vi "RW_Module.vi"(7 "N_modules":i32, 8 "error in":errorcluster, 9 "RD_WR param":T1, 10 "Data Reference":T2, 11 "Status Reference":T3) -> (0 "error out":errorcluster, 1 "stopped":bool)   [LabVIEW 2019, in "MB_TCP1.lvlib"]
uses:
  MB_TCP1.lvlib
  ICPCON Status/Ctl/ICPCON Status.ctl
  ICPCON Registers/Ctl/ICPCON Data.ctl
  ICPCON Param/ICPCON Param.ctl
  MB_TCP_NS300.vi
  MB_TCP_7016i.vi
  MB_TCP_7051.vi
  MB_TCP_7024i.vi
  MB_TCP_7018o.vi
  MB_TCP_7018.vi
  MB_TCP_7018i.vi
  MB_TCP_7017.vi
  MB_TCP_ZERO.vi
  ICPCON Status/ICPCON Status.lvlib
  ICPCON Registers/ICPCON Registers.lvlib
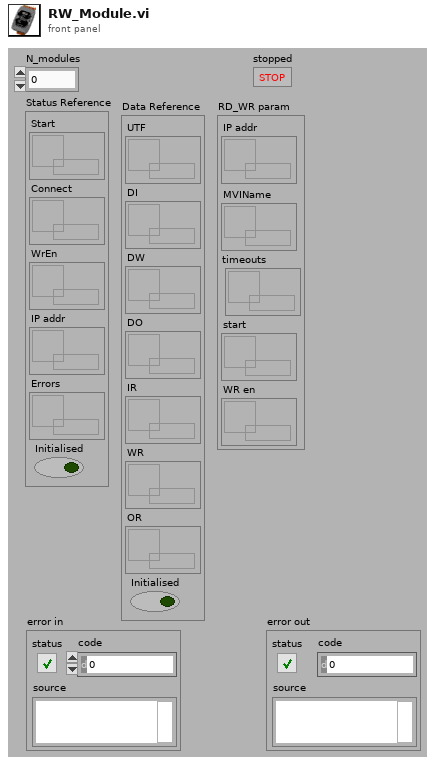
[diagram p1: front panel]
types:
  T1 = typedef "ICPCON Param.ctl" = cluster{"IP addr":refnum<data-value>, "MVIName":refnum<data-value>, "timeouts":refnum<data-value>, "start":refnum<data-value>, "WR en":refnum<data-value>}
  T2 = typedef "ICPCON Registers.lvlib/ICPCON Data.ctl" = cluster{"UTF":refnum<data-value>, "DI":refnum<data-value>, "DW":refnum<data-value>, "DO":refnum<data-value>, "IR":refnum<data-value>, "WR":refnum<data-value>, "OR":refnum<data-value>, "Initialised":bool}
  T3 = typedef "ICPCON Status.lvlib/ICPCON Status.ctl" = cluster{"Start":refnum<data-value>, "Connect":refnum<data-value>, "WrEn":refnum<data-value>, "IP addr":refnum<data-value>, "Errors":refnum<data-value>, "Initialised":bool}
  T4 = enum16{"initialize", "call modules", "work", "stop modules", "standby"}
  T5 = enum32{"Bad", "Idle", "Run top level", "Running"}
  T6 = cluster{"Remote IP Address":string, "Remote Port":u16}[]
  T7 = cluster{"conn_timeout":i32, "reconn_timeout":i32, "N attempt max":i32, "t_reset_TTL":i32, "write_timeout":i32, "read_timeout":i32, "period":i32}[]
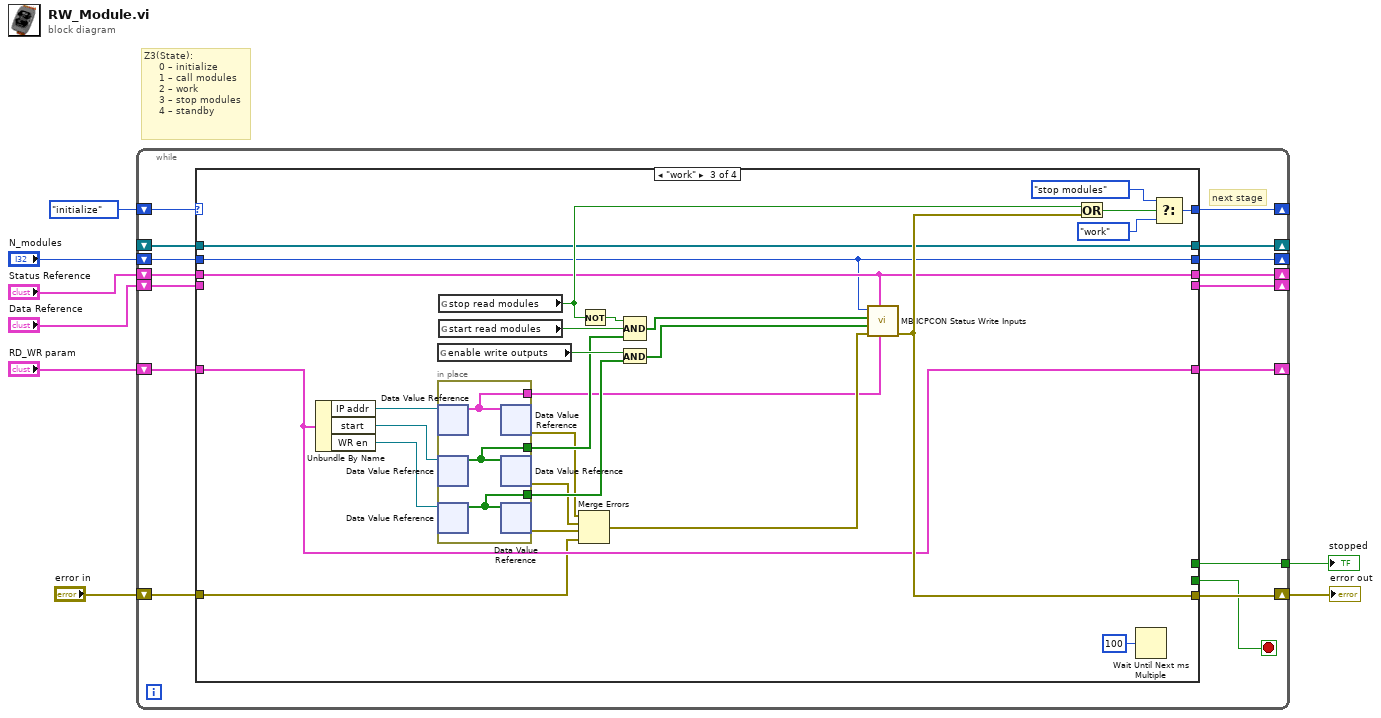
[diagram p0: block diagram]
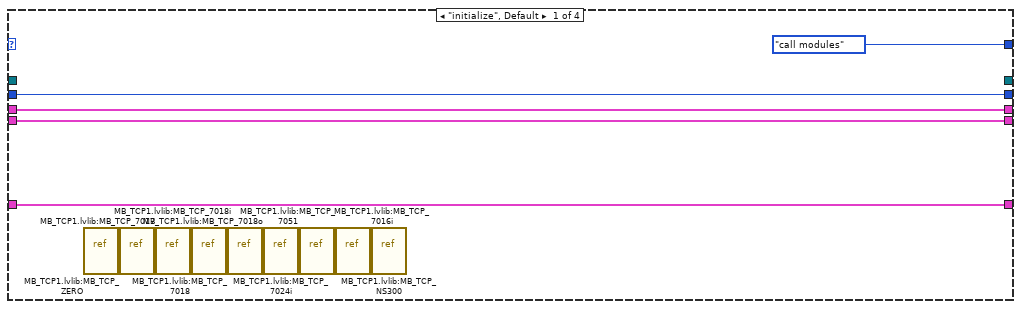
[diagram p2: hidden frame]
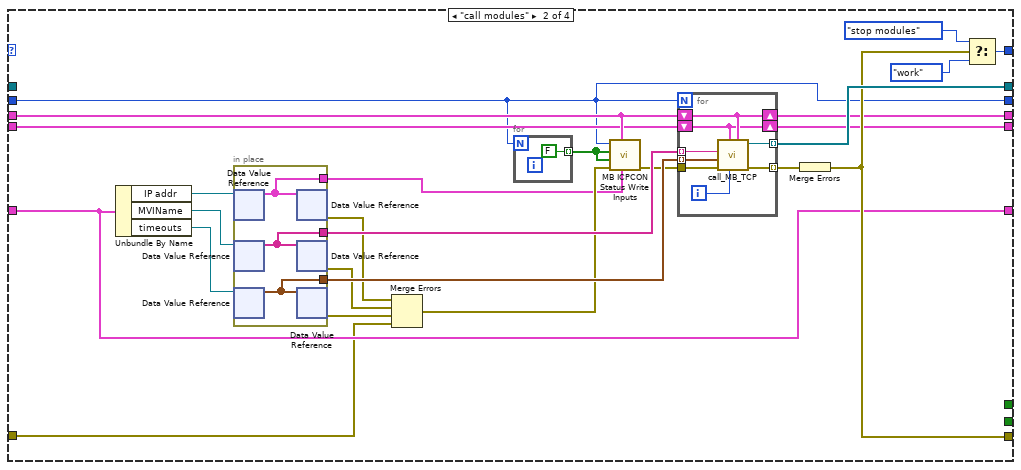
[diagram p3: hidden frame]
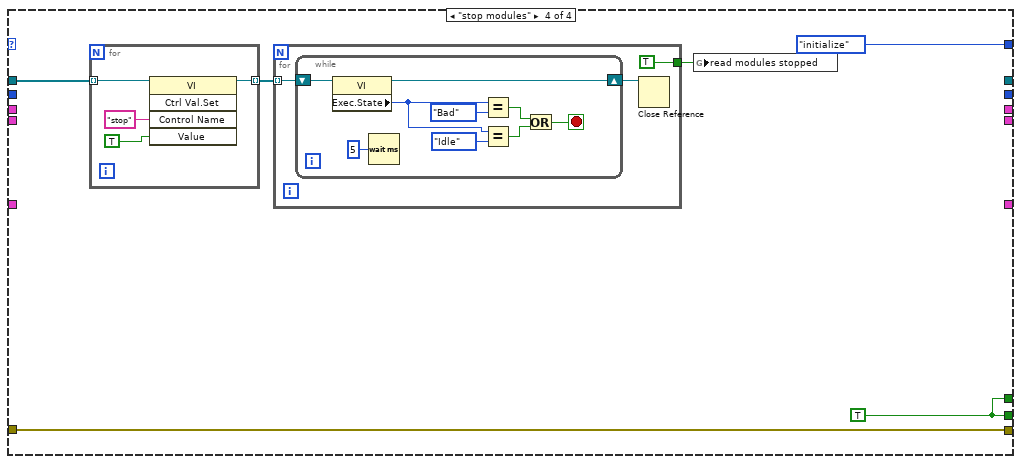
[diagram p4: hidden frame]
diagram:
  # "Z3(State):\n     0 – initialize \n     1 – call modules\n     2 – work\n     3 – stop modules\n     4 – standby"
  n1 = while {
    shift-right: [w24] -> _
    shift-left: T4."initialize" -> [w22]
    shift-right: [w23] -> _
    shift-left: _ -> [w21]
    shift-right: [w20] -> w7
    shift-left: "error in" -> [w19]
    tunnel: [w18] -> w6
    shift-right: [w9] -> _
    shift-left: "N_modules" -> [w16]
    shift-right: [w11] -> _
    shift-left: "Status Reference" -> [w14]
    shift-right: [w10] -> _
    shift-left: "Data Reference" -> [w15]
    shift-right: [w12] -> _
    shift-left: "RD_WR param" -> [w13]
    stop <- w17 stop-if-true
    # "next stage"
    n2 = case shown="\"work\"" w22 {
      tunnel: [T4."call modules" w42 w86 T4."initialize"] -> w24
      tunnel: w16 -> [w28 w31 w74 _]
      tunnel: w14 -> [w27 w49 w75 _]
      tunnel: w15 -> [w26 w48 _ _]
      tunnel: [_ w46 w81 _] -> w23
      tunnel: w21 -> [_ _ w81 w100]
      tunnel: [_ w41 w83 w99] -> w20
      tunnel: w19 -> [_ w33 w69 w99]
      tunnel: [_ _ _ w98] -> w18
      tunnel: [_ _ _ w98] -> w17
      tunnel: w13 -> [w25 w38 w76 _]
      tunnel: [w25 w38 w76 _] -> w12
      tunnel: [w27 w40 w75 _] -> w11
      tunnel: [w26 w39 _ _] -> w10
      tunnel: [w28 w31 w74 _] -> w9
      frame "initialize", Default {
        n3 = vi-ref "MB_TCP1.lvlib:MB_TCP_ZERO.vi"() -> ()  [unwired: 1 out]
        n4 = vi-ref "MB_TCP1.lvlib:MB_TCP_7017.vi"() -> ()  [unwired: 1 out]
        n5 = vi-ref "MB_TCP1.lvlib:MB_TCP_7018i.vi"() -> ()  [unwired: 1 out]
        n6 = vi-ref "MB_TCP1.lvlib:MB_TCP_7018.vi"() -> ()  [unwired: 1 out]
        n7 = vi-ref "MB_TCP1.lvlib:MB_TCP_7018o.vi"() -> ()  [unwired: 1 out]
        n8 = vi-ref "MB_TCP1.lvlib:MB_TCP_7024i.vi"() -> ()  [unwired: 1 out]
        n9 = vi-ref "MB_TCP1.lvlib:MB_TCP_7051.vi"() -> ()  [unwired: 1 out]
        n10 = vi-ref "MB_TCP1.lvlib:MB_TCP_7016i.vi"() -> ()  [unwired: 1 out]
        n11 = vi-ref "MB_TCP1.lvlib:MB_TCP_NS300.vi"() -> ()  [unwired: 1 out]
      }
      frame "call modules" {
        n12 = Unbundle By Name(w38) -> ("IP addr"=w45:refnum<data-value>, "MVIName"=w47:refnum<data-value>, "timeouts"=w37:refnum<data-value>)
        n13 = in-place {
          in-place-border: [w65] -> w30
          in-place-border: [w64] -> w54
          in-place-border: [w63] -> w53
          n14 = in-place-dvr #1(w45) -> (w65:T6)  [unwired: 1 out]
          n15 = in-place-dvr #2(w47) -> (w64:string[])  [unwired: 1 out]
          n16 = in-place-dvr #3(w37) -> (w63:T7)  [unwired: 1 out]
          n17 = in-place-dvr #1(w65) -> (w36:errorcluster)  [unwired: 1 out]
          n18 = in-place-dvr #2(w64) -> (w35:errorcluster)  [unwired: 1 out]
          n19 = in-place-dvr #3(w63) -> (w34:errorcluster)  [unwired: 1 out]
        }
        n20 = Merge Errors(w36, w35, w34, w33) -> (w32:errorcluster)
        n21 = for {
          N: w31 -> [_]
          tunnel: [FALSE ("Write Enable")] -> w52 mode=indexing
        }
        n22 = call "MB ICPCON Status Write Inputs.vi"("IP address"=w30, "Status Reference"=w49, "error in (no error)"=w32, "Write Enable"=w52, "Start"=w52, "Lenght"=w31) -> ("error out"=w51:errorcluster)  [unwired: 5 in]
        n23 = for {
          N: w31 -> [_]
          tunnel: [w62] -> w50 mode=indexing
          tunnel: w53 -> [w60] mode=indexing
          tunnel: [w61] -> w46 mode=indexing
          tunnel: w54 -> [w59] mode=indexing
          tunnel: w51 -> [w57]
          shift-right: [w56] -> w40
          shift-left: w49 -> [w56]
          shift-right: [w55] -> w39
          shift-left: w48 -> [w55]
          i -> [w58]
          n24 = call "call_MB_TCP.vi"("Status Reference"=w56, "N"=w58, "Data Reference"=w55, "error in"=w57, "timeouts"=w60, "Module Name"=w59) -> ("error out"=w62:errorcluster, "vi reference"=w61:refnum<vi>)  [unwired: 4 in]
        }
        n25 = Merge Errors(w50) -> (w41:errorcluster)
        n26 = Select(t=T4."stop modules", s=w41, f=T4."work") -> (s? t:f=w42:T4)
      }
      frame "work" {
        n27 = Unbundle By Name(w76) -> ("IP addr"=w78:refnum<data-value>, "start"=w73:refnum<data-value>, "WR en"=w77:refnum<data-value>)
        n28 = global read "az_parameters_200121.vi" "enable write outputs"() -> (w89:bool)
        n29 = in-place {
          in-place-border: [w96] -> w67
          in-place-border: [w95] -> w88
          in-place-border: [w94] -> w87
          n30 = in-place-dvr #4(w78) -> (w96:T6)  [unwired: 1 out]
          n31 = in-place-dvr #5(w73) -> (w95:bool[])  [unwired: 1 out]
          n32 = in-place-dvr #6(w77) -> (w94:bool[])  [unwired: 1 out]
          n33 = in-place-dvr #4(w96) -> (w72:errorcluster)  [unwired: 1 out]
          n34 = in-place-dvr #5(w95) -> (w71:errorcluster)  [unwired: 1 out]
          n35 = in-place-dvr #6(w94) -> (w70:errorcluster)  [unwired: 1 out]
        }
        n36 = global read "az_parameters_200121.vi" "stop read modules"() -> (w85:bool)
        n37 = global read "az_parameters_200121.vi" "start read modules"() -> (w90:bool)
        n38 = Merge Errors(w72, w71, w70, w69) -> (w68:errorcluster)
        n39 = Not(x=w85) -> (.not. x?=w93:bool)
        n40 = And(x=w89, y=w87) -> (x .and. y?=w92:bool[])
        n41 = Compound Arithmetic op=AND(w93, w90, w88) -> (w91:bool[])
        n42 = call "MB ICPCON Status Write Inputs.vi"("IP address"=w67, "Status Reference"=w75, "error in (no error)"=w68, "Write Enable"=w92, "Start"=w91, "Lenght"=w74) -> ("error out"=w83:errorcluster)  [unwired: 5 in]
        n43 = Or(x=w85, y=w83) -> (x .or. y?=w84:bool)
        n44 = Wait Until Next ms Multiple(millisecond multiple=u32 100) -> ()  [unwired: 1 out]
        n45 = Select(t=T4."stop modules", s=w84, f=T4."work") -> (s? t:f=w86:T4)
      }
      frame "stop modules" {
        w98 = TRUE
        n46 = for {
          tunnel: w100 -> [w117] mode=indexing
          tunnel: [w116] -> w102 mode=indexing
          n47 = invoke class="VI" method="Ctrl Val.Set"(reference=w117, "Control Name"="stop", "Value"=TRUE) -> (reference out=w116:refnum<vi>)  [unwired: 2 in, 4 out]
        }
        n48 = for {
          tunnel: w102 -> [w105] mode=indexing
          tunnel: [TRUE ("read modules stopped")] -> w101
          n49 = while {
            shift-right: [w113] -> w103
            shift-left: w105 -> [w114]
            stop <- w107 stop-if-true
            n50 = property class="VI"(reference=w114) -> (reference out=w113:refnum<vi>, "Exec.State"=w108:T5)  [unwired: 1 in, 1 out]
            n51 = Wait (ms)(milliseconds to wait=u32 5) -> ()  [unwired: 1 out]
            n52 = Equal?(x=w108, y=T5."Bad") -> (x = y?=w111:bool)
            n53 = Equal?(x=w108, y=T5."Idle") -> (x = y?=w106:bool)
            n54 = Or(x=w111, y=w106) -> (x .or. y?=w107:bool)
          }
          n55 = Close Reference(reference=w103) -> ()  [unwired: 1 in, 1 out]
        }
        n56 = global write "az_parameters_200121.vi" "read modules stopped"(w101) -> ()
      }
    }
  }
  "error out" <- w7
  "stopped" <- w6
